vi "Snap Picture.vi"(6 "Image In":T2, 7 "Session In":T1) -> (2 "Image out":T2)   [LabVIEW 2011]
uses:
  <vilib>/vision/Image Controls.llb/IMAQ Image.ctl
  <vilib>/userDefined/High Color/IMAQdx.ctl
  <vilib>/vision/driver/NI_Vision_Acquisition_Software.lvlib
  <vilib>/vision/NI_Vision_Development_Module.lvlib
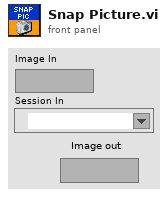
[diagram p1: front panel]
types:
  T1 = typedef "IMAQdx.ctl" = refnum<k21>
  T2 = typedef "IMAQ Image.ctl" = refnum<image>
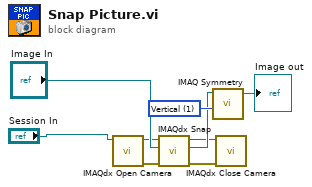
[diagram p0: block diagram]
diagram:
  w9 = u32 1 items=["Horizontal", "Vertical", "Central", "1st Diagonal", "2nd Diagonal"] ("Type of Symmetry")
  n1 = call <vilib>:"IMAQdx Open Camera.vi"("Session In"="Session In") -> ("error out"=w5:errorcluster, "Session Out"=w4:T1)  [unwired: 9 in]
  n2 = call <vilib>:"IMAQdx Snap.vi"("error in"=w5, "Image In"="Image In", "Session In"=w4) -> ("error out"=w2:errorcluster, "Image Out"=w8:T2, "Session Out"=w1:T1)  [unwired: 6 in]
  n3 = call "IMAQ Symmetry"("Type of Symmetry"=w9, "Image Src"=w8) -> ("Image Dst Out"=→"Image out":T2)  [unwired: 3 in, 1 out]
  n4 = call <vilib>:"IMAQdx Close Camera.vi"("error in"=w2, "Session In"=w1) -> ()  [unwired: 9 in, 1 out]
